vi "InitPreferences.vi"(8 "error in (no error)":errorcluster, 11 "Preferences in":refnum<class "SetListPrefs.lvclass">) -> (0 "error out":errorcluster, 2 "Raw XML":string, 3 "Preferences out":refnum<class "SetListPrefs.lvclass">)   [LabVIEW 2013, in "SetListPrefs.lvclass"]
uses:
  SetListPrefs.lvclass
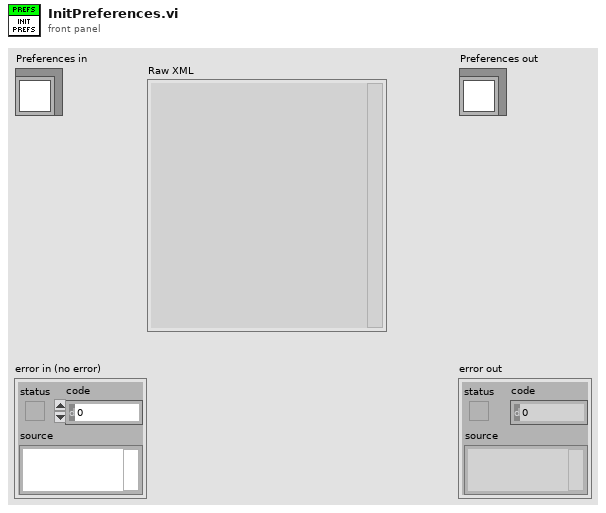
[diagram p1: front panel]
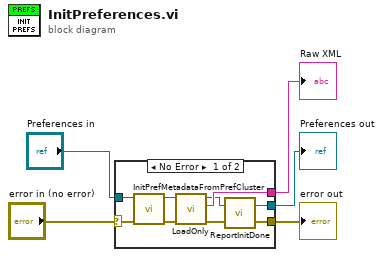
[diagram p0: block diagram]
diagram:
  n1 = case shown="No Error" "error in (no error)" {
    selector: "error in (no error)" -> [w13 w16]
    tunnel: [w8 w16] -> w4
    tunnel: [w6 w15] -> w2
    tunnel: "Preferences in" -> [w14 w15]
    tunnel: [w10 _] -> w1
    frame No Error {
      n2 = call "InitPrefMetadataFromPrefCluster.vi"("error in (no error)"=w13, "Preferences in"=w14) -> ("error out"=w12:errorcluster, "Preferences out"=w11:refnum<class "SetListPrefs.lvclass">)  [unwired: 8 in]
      n3 = call "LoadOnly.vi"("error in (no error)"=w12, "Preferences in"=w11) -> ("error out"=w9:errorcluster, "Raw XML"=w10:string, "Preferences out"=w7:refnum<class "SetListPrefs.lvclass">)  [unwired: 7 in]
      n4 = call "ReportInitDone.vi"("error in (no error)"=w9, "Preferences in"=w7) -> ("error out"=w8:errorcluster, "Preferences out"=w6:refnum<class "SetListPrefs.lvclass">)
    }
    frame Error {
    }
  }
  "error out" <- w4
  "Preferences out" <- w2
  "Raw XML" <- w1
